vi "SetAutoLEDs.vi"(1 "AvailableRoutines":T1, 2 "AutoStartingPosition":T7) -> ()   [LabVIEW 2017]
uses:
  Autonomous/TypeDef/AutoStartingPositions.ctl
  Autonomous/TypeDef/AutoRoutineSet.ctl
  Autonomous/TypeDef/AutoStep.ctl
  Autonomous/TypeDef/AutoWaypointType.ctl
  Pathfinder/Pathfinder-LabVIEW/Pathfinder-Lib/VIs/Waypoint.ctl
  Implements/Arm/TypeDefs/ArmTargetPosition.ctl
  Implements/TypeDefs/IntakeState.ctl
  TypeDefs/LEDAutoMode.ctl
  0656a6c4-feae-4b02-aaa5-f0e9803bc6a1.vi
  Global_Var-RefNum/LEDData.vi
  Pathfinder/Pathfinder-LabVIEW/Pathfinder-Lib/Pathfinder.lvlib
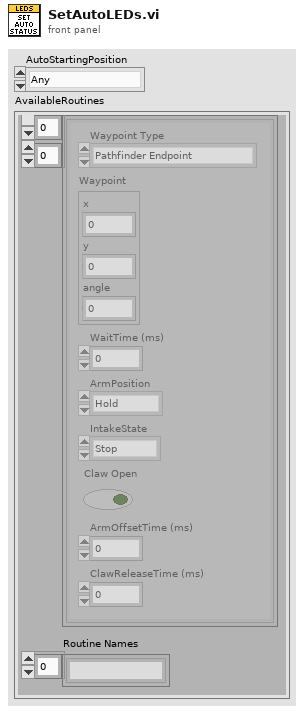
[diagram p1: front panel]
types:
  T1 = typedef "AutoRoutineSet.ctl" = cluster{"Routines":T2[][], "Routine Names":string[]}
  T2 = typedef "AutoStep.ctl" = cluster{"Waypoint Type":T3, "Waypoint":T4, "WaitTime (ms)":u16, "ArmPosition":T5, "IntakeState":T6, "Claw Open":bool, "ArmOffsetTime (ms)":u16, "ClawReleaseTime (ms)":i32}
  T3 = typedef "AutoWaypointType.ctl" = enum16{"Pathfinder Endpoint", "Pathfinder Waypoint", "Zero-Radius Turn Endpoint", "Stationary", "Vision Assist Endpoint", "Stop"}
  T4 = typedef "Pathfinder.lvlib/Waypoint.ctl" = cluster{"x":dbl, "y":dbl, "angle":dbl}
  T5 = typedef "ArmTargetPosition.ctl" = enum16{"Hold", "Switch", "Scale Low", "Scale High", "Climb", "Back Place"}
  T6 = typedef "IntakeState.ctl" = enum16{"Stop", "Forward", "Reverse", "Forward Open"}
  T7 = typedef "AutoStartingPositions.ctl" = enum16{"Any", "Left", "Center", "Right"}
  T8 = typedef "LEDAutoMode.ctl" = enum16{"Auto Left Switch", "Auto Left Scale", "Auto Center Switch", "Auto Center Scale", "Auto Right Switch", "Auto Right Scale", "Auto Line"}
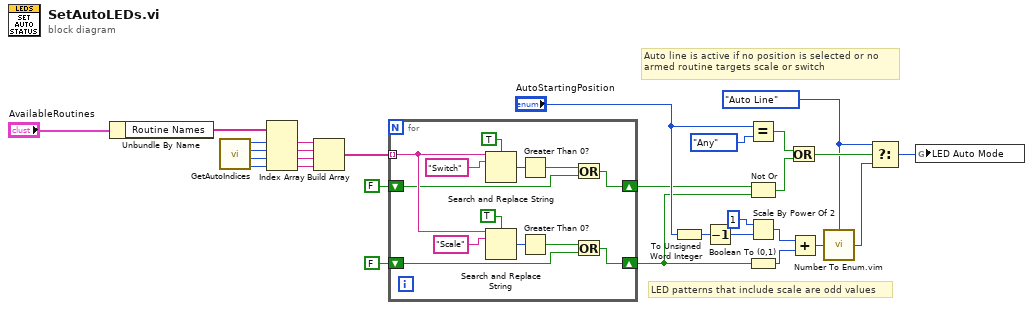
[diagram p0: block diagram]
diagram:
  w4 = LEDAutoMode."Auto Line" ("LED Auto Mode")
  # "Auto line is active if no position is selected or no\narmed routine targets scale or switch"
  # "LED patterns that include scale are odd values"
  n1 = Unbundle By Name("AvailableRoutines") -> ("Routine Names"=w28:string[])
  n2 = call "GetAutoIndices.vi"() -> ("LLL Routine Index"=w27:u16, "LRL Routine Index"=w26:u16, "RLR Routine Index"=w25:u16, "RRR Routine Index"=w24:u16)  [unwired: 1 in]
  n3 = Index Array(array=w28, index #1=w27, index #2=w26, index #3=w25, index #4=w24) -> (element #1=w23:string, element #2=w22:string, element #3=w21:string, element #4=w20:string)
  n4 = Build Array(w23, w22, w21, w20) -> (w19:string[])
  n5 = for {
    tunnel: w19 -> [w36] mode=indexing
    shift-right: [w34] -> w9
    shift-left: FALSE -> [w33]
    shift-right: [w31] -> w1
    shift-left: FALSE -> [w30]
    n6 = Search and Replace String(case sensitive?=TRUE ("ignore case? (F)"), input string=w36, search string="Switch") -> (number of replacements=w41:i32)  [unwired: 5 in, 3 out]
    n7 = Search and Replace String(case sensitive?=TRUE ("ignore case? (F)"), input string=w36, search string="Scale") -> (number of replacements=w38:i32)  [unwired: 5 in, 3 out]
    n8 = Greater Than 0?(x=w41) -> (x > 0?=w35:bool)
    n9 = Greater Than 0?(x=w38) -> (x > 0?=w32:bool)
    n10 = Or(x=w35, y=w33) -> (x .or. y?=w34:bool)
    n11 = Or(x=w32, y=w30) -> (x .or. y?=w31:bool)
  }
  n12 = To Unsigned Word Integer(number="AutoStartingPosition") -> (unsigned 16bit integer=w6:u16)
  n13 = Decrement(x=w6) -> (x-1=w10:u16)
  n14 = Equal?(x="AutoStartingPosition", y=AutoStartingPositions."Any" ("AutoStartingPosition")) -> (x = y?=w15:bool)
  n15 = Not Or(1:w1, 2:w9) -> (0:w14:bool)
  n16 = Scale By Power Of 2(n=i16 1, x=w10) -> (x*2^n=w8:u16)
  n17 = Boolean To (0,1)(Boolean=w1) -> (0, 1=w7:i16)
  n18 = Or(x=w15, y=w14) -> (x .or. y?=w13:bool)
  n19 = Add(x=w8, y=w7) -> (x+y=w3:u16)
  n20 = call "Number To Enum.vim"("number"=w3, "enum type"=w4) -> ("number as enum"=w5:T8)
  n21 = Select(t=w4, s=w13, f=w5) -> (s? t:f=w2:T8)
  n22 = global write "LEDData.vi" "LED Auto Mode"(w2) -> ()
